vi "Circular Buffer Timestamp subVI.vi"(6 "History Length [1024]":i32, 7 "reset":bool, 10 "Buffer in":waveform(dbl), 11 "Waveform in in":waveform(dbl)) -> (2 "Buffer out":waveform(dbl), 3 "Waveform out":waveform(dbl))   [LabVIEW 2019, in "xy_utilities.lvlib"]
uses:
  xy_utilities.lvlib
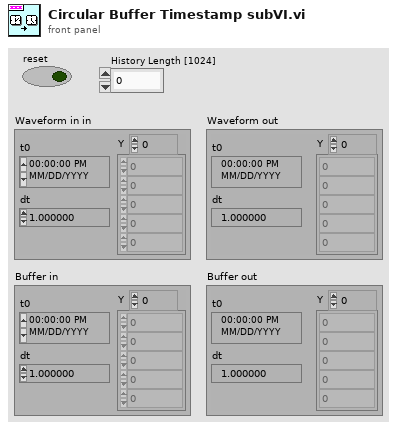
[diagram p1: front panel]
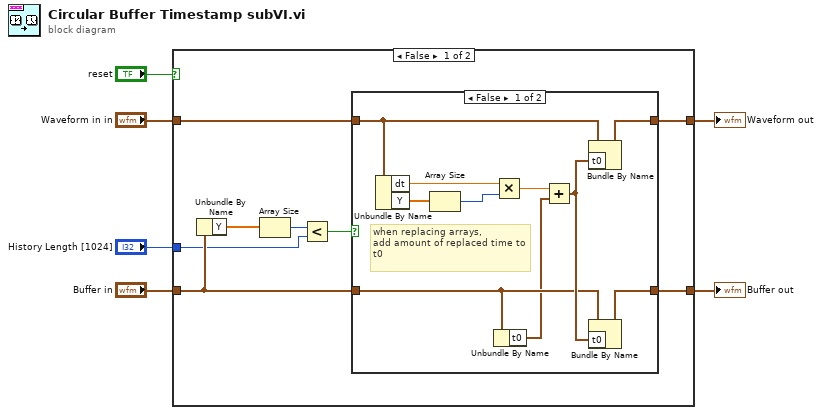
[diagram p0: block diagram]
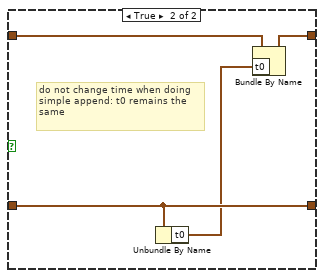
[diagram p2: hidden frame]
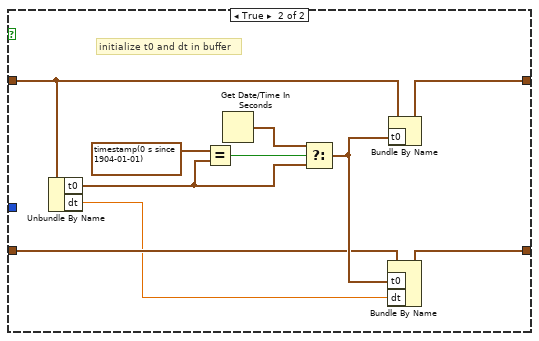
[diagram p3: hidden frame]
diagram:
  n1 = case shown="False" "reset" {
    tunnel: "Buffer in" -> [w11 w31]
    tunnel: [w9 w30] -> w3
    tunnel: "Waveform in in" -> [w8 w34]
    tunnel: [w7 w32] -> w5
    tunnel: "History Length [1024]" -> [w10 _]
    frame False {
      n2 = Unbundle By Name(w11) -> ("Y"=w14:dbl[])
      n3 = Array Size(array=w14) -> (size(s)=w13:i32)
      n4 = Less?(x=w13, y=w10) -> (x < y?=w12:bool)
      n5 = case shown="False" w12 {
        tunnel: [w21 w28] -> w9
        tunnel: w11 -> [w18 w28]
        tunnel: w8 -> [w15 w27]
        tunnel: [w20 w26] -> w7
        frame False {
          # "when replacing arrays,\nadd amount of replaced time to t0"
          n6 = Unbundle By Name(w15) -> ("dt"=w24:dbl, "Y"=w23:dbl[])
          n7 = Array Size(array=w23) -> (size(s)=w22:i32)
          n8 = Multiply(x=w24, y=w22) -> (x*y=w17:dbl)
          n9 = Unbundle By Name(w18) -> ("t0"=w16:timestamp)
          n10 = Add(x=w17, y=w16) -> (x+y=w19:timestamp)
          n11 = Bundle By Name(cluster=w15, "t0"=w19) -> (w20:waveform(dbl))
          n12 = Bundle By Name(cluster=w18, "t0"=w19) -> (w21:waveform(dbl))
        }
        frame True {
          # "do not change time when doing simple append: t0 remains the same"
          n13 = Unbundle By Name(w28) -> ("t0"=w25:timestamp)
          n14 = Bundle By Name(cluster=w27, "t0"=w25) -> (w26:waveform(dbl))
        }
      }
    }
    frame True {
      # "initialize t0 and dt in buffer"
      n15 = Unbundle By Name(w34) -> ("t0"=w36:timestamp, "dt"=w29:dbl)
      n16 = Equal?(x=timestamp(0 s since 1904-01-01), y=w36) -> (x = y?=w37:bool)
      n17 = Get Date/Time In Seconds() -> (seconds since 1Jan1904=w35:timestamp)
      n18 = Select(t=w35, s=w37, f=w36) -> (s? t:f=w33:timestamp)
      n19 = Bundle By Name(cluster=w31, "t0"=w33, "dt"=w29) -> (w30:waveform(dbl))
      n20 = Bundle By Name(cluster=w34, "t0"=w33) -> (w32:waveform(dbl))
    }
  }
  "Waveform out" <- w5
  "Buffer out" <- w3
